vi "Untitled 2.vi"() -> ()   [LabVIEW 2024]
uses:
  CANopen/CANopen.lvclass
  HAL/HAL/Devices/CAN Interfaces/PCAN/PCAN.lvclass
  HAL/HAL/Configurations/CFG Base/CFG Base.lvclass
panel:
  in  "Start Heartbeats":bool
  out "Service Map":map{string, u8[]}(c390)
  out "Heartbeats":T1(c390)
  out "Emergency":bool
  in  "stop":bool
  out "error out":errorcluster
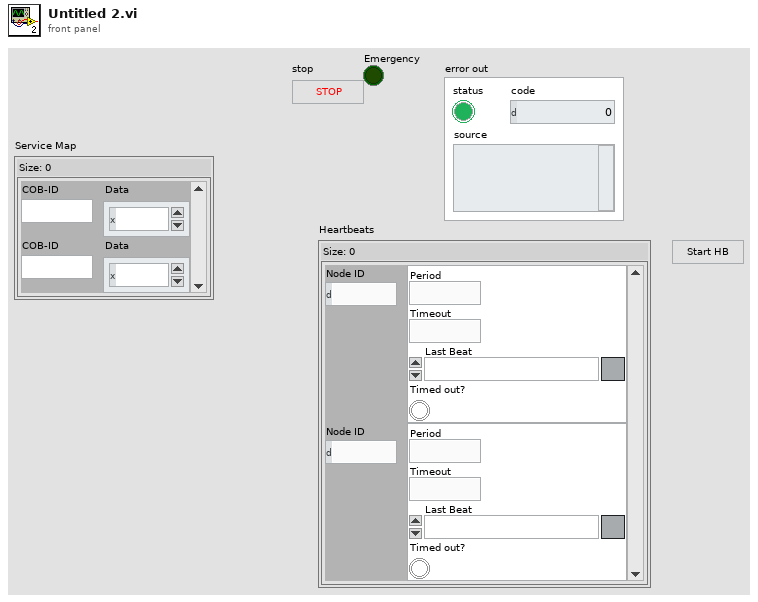
[diagram p1: front panel]
types:
  T1 = map{u8, cluster{"Period":u16, "Timeout":u16, "Last Beat":timestamp, "Timed out?":bool}}
  T2 = map{u8, cluster{"Period":u16, "Timeout":u16, "Last Beat":timestamp, "Timed Out?":bool}}
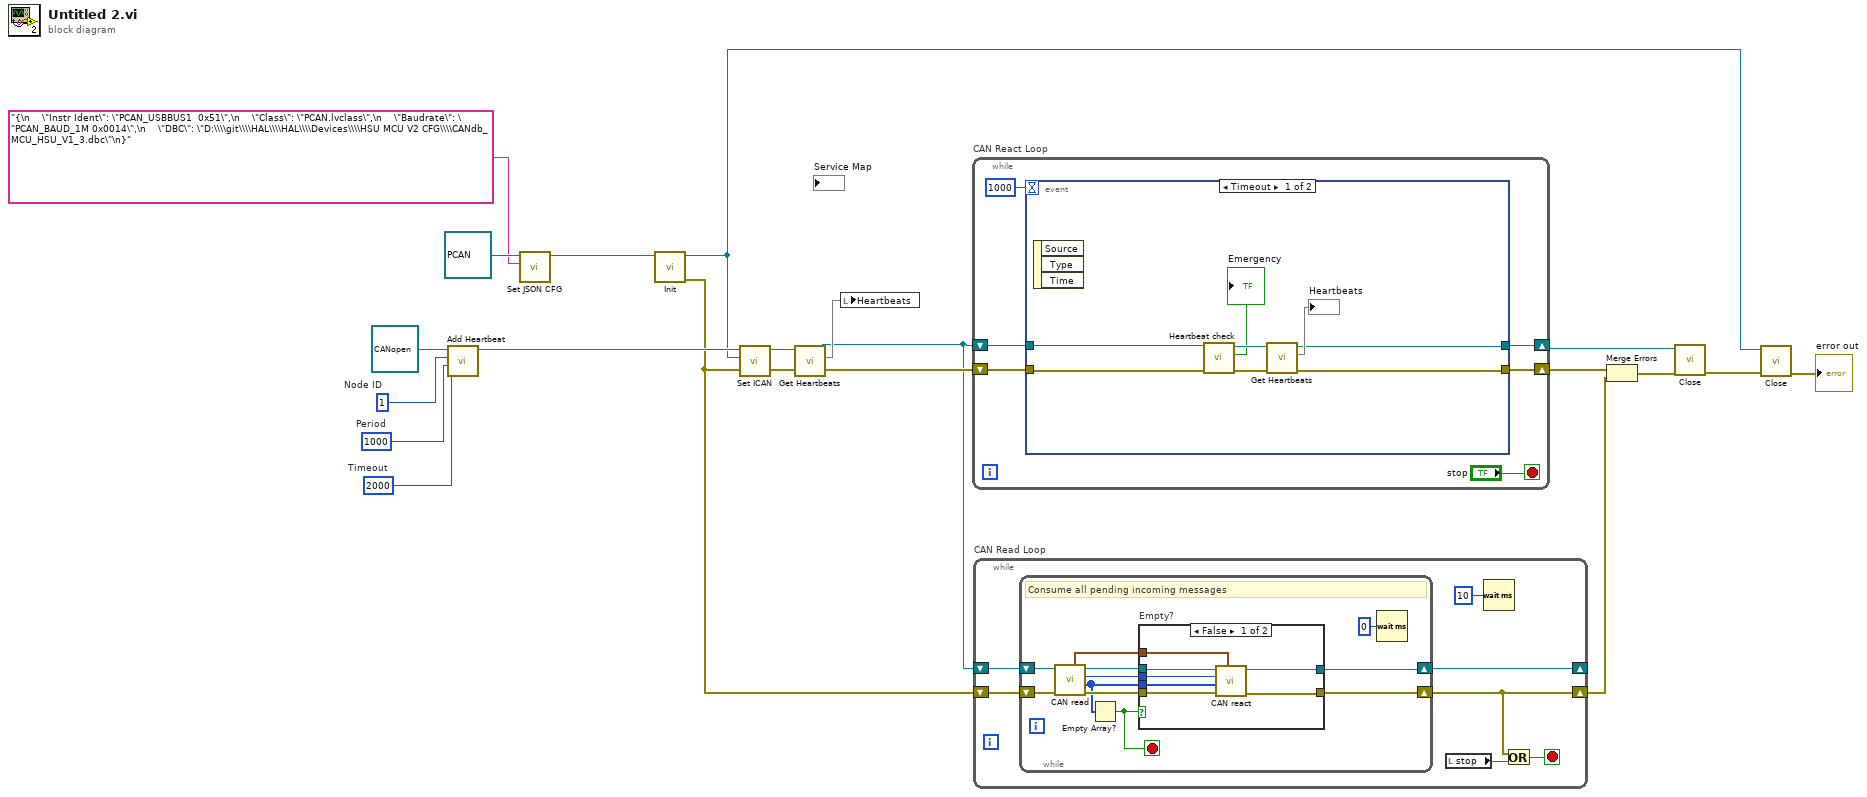
[diagram p0: block diagram]
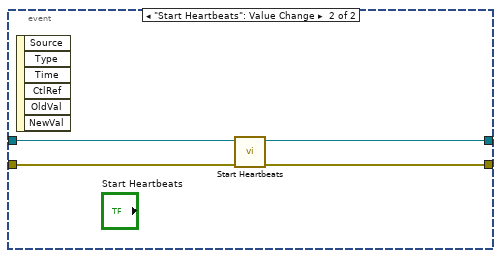
[diagram p2: hidden frame]
diagram:
  w10 = u16 2000  # Timeout
  w11 = u16 1000  # Period
  w12 = u8 1  # Node ID
  n1 = call "Add Heartbeat.vi"("Timeout"=w10, "Period"=w11, "Node ID"=w12, "CANopen in"=refnum<class "CANopen.lvclass"> refnum ("canopen.lvlib:CANopen.lvclass")) -> ("CANopen out"=w15:refnum<class "CANopen.lvclass">)  [unwired: 7 in]
  n2 = call "Set JSON CFG.vi"("<JSON>CFG"="{\n    \"Instr Ident\": \"PCAN_USBBUS1  0x51\",\n    \"Class\": \"PCAN.lvclass\",\n    \"Baudrate\": \"PCAN_BAUD_1M 0x0014\",\n    \"DBC\": \"D:\\\\git\\\\HAL\\\\HAL\\\\Devices\\\\HSU MCU V2 CFG\\\\CANdb_MCU_HSU_V1_3.dbc\"\n}", "CFG Base in"=refnum<class "PCAN.lvclass"> refnum ("PCAN.lvclass")) -> ("CFG Base out"=w17:refnum<class "PCAN.lvclass">)  [unwired: 9 in]
  n3 = call-dynamic "Init.vi"("PCAN in"=w17) -> ("error out"=w6:errorcluster, "PCAN out"=w13:refnum<class "PCAN.lvclass">)  [unwired: 9 in]
  n4 = call "Set ICAN.vi"("ICAN"=w13, "CANopen in"=w15) -> ("CANopen out"=w5:refnum<class "CANopen.lvclass">)  [unwired: 9 in]
  n5 = call "Get Heartbeats.vi"("CANopen in"=w5) -> ("Heartbeats"=w7:T2, "CANopen out"=w4:refnum<class "CANopen.lvclass">)  [unwired: 9 in]
  n6 = local write "Heartbeats"(w7) -> ()
  n7 = while "CAN React Loop" {
    shift-right: [w22] -> w8
    shift-left: w6 -> [w25]
    shift-right: [w23] -> w1
    shift-left: w4 -> [w24]
    stop <- "stop" stop-if-true
    n8 = event shown="[0] Timeout" {
      selector: _ -> [_ _]
      dyn-events: _ -> [_ _]
      timeout: 1000 -> [_ _]
      tunnel: w25 -> [w29 w36]
      tunnel: w24 -> [w28 w34]
      tunnel: [w26 w33] -> w23
      tunnel: [w27 w35] -> w22
      event Timeout {
        n9 = event-data() -> ()  [unwired: 1 in, 3 out]
        n10 = call "Heartbeat check.vi"("error in"=w29, "CANopen in"=w28) -> ("error out"=w27:errorcluster, "Emergency"=→"Emergency":bool, "CANopen out"=w32:refnum<class "CANopen.lvclass">)  [unwired: 7 in]
        n11 = call "Get Heartbeats.vi"("CANopen in"=w32) -> ("Heartbeats"=→"Heartbeats":T2, "CANopen out"=w26:refnum<class "CANopen.lvclass">)  [unwired: 9 in]
      }
      event "Start Heartbeats": Value Change {
        n12 = event-data() -> ()  [unwired: 1 in, 6 out]
        n13 = call "Start Heartbeats.vi"("error in"=w36, "CANopen in"=w34) -> ("error out"=w35:errorcluster, "CANopen out"=w33:refnum<class "CANopen.lvclass">)  [unwired: 8 in]
      }
    }
  }
  n14 = while "CAN Read Loop" {
    shift-right: [w40] -> w9
    shift-left: w6 -> [w43]
    shift-right: [w39] -> _
    shift-left: w4 -> [w42]
    stop <- w41 stop-if-true
    n15 = while {
      shift-right: [w51] -> w40
      shift-left: w43 -> [w54]
      shift-right: [w44] -> w39
      shift-left: w42 -> [w53]
      stop <- w48 stop-if-true
      # "Consume all pending incoming messages"
      n16 = call "CAN read.vi"("error in"=w54, "CANopen in"=w53) -> ("error out"=w50:errorcluster, "Data"=w49:u8[], "COB-ID"=w52:u32, "CANopen out"=w45:refnum<class "CANopen.lvclass">, "Time Stamp"=w47:timestamp)  [unwired: 5 in]
      n17 = Empty Array?(array=w49) -> (empty?=w48:bool)
      n18 = case "Empty?" shown="False" w48 {
        tunnel: w52 -> [w57 _]
        tunnel: w49 -> [w56 _]
        tunnel: [w60 w63] -> w51
        tunnel: w50 -> [w61 w63]
        tunnel: w47 -> [w55 _]
        tunnel: w45 -> [w59 w62]
        tunnel: [w58 w62] -> w44
        frame False {
          n19 = call "CAN react.vi"("Time Stamp"=w55, "error in"=w61, "Data"=w56, "COB-ID"=w57, "CANopen in"=w59) -> ("error out"=w60:errorcluster, "CANopen out"=w58:refnum<class "CANopen.lvclass">)  [unwired: 5 in]
        }
        frame True {
        }
      }
      n20 = Wait (ms)(milliseconds to wait=u32 0) -> ()  [unwired: 1 out]
    }
    n21 = local read "stop"() -> (w37:bool)
    n22 = Wait (ms)(milliseconds to wait=10) -> ()  [unwired: 1 out]
    n23 = Or(x=w40, y=w37) -> (x .or. y?=w41:bool)
  }
  n24 = Merge Errors(w8, w9) -> (w3:errorcluster)
  n25 = call "Close.vi"("error in"=w3, "CANopen in"=w1) -> ("error out"=w2:errorcluster)  [unwired: 8 in, 1 out]
  n26 = call-dynamic "Close.vi"("error in"=w2, "PCAN in"=w13) -> ("error out"=→"error out":errorcluster)  [unwired: 8 in, 1 out]
